vi "SubPanel_VIsList.vi"(8 "error in (no error)":errorcluster, 11 "SubPanelPath in":path) -> (0 "error out":errorcluster, 1 "SubP_VIsPathList":path[](array[path]), 2 "SubPanelsVis":string[](array[string]), 3 "SubPanelPath out":path)   [LabVIEW 2014, in "SubPanelModule.lvlib"]
uses:
  SubPanelModule.lvlib
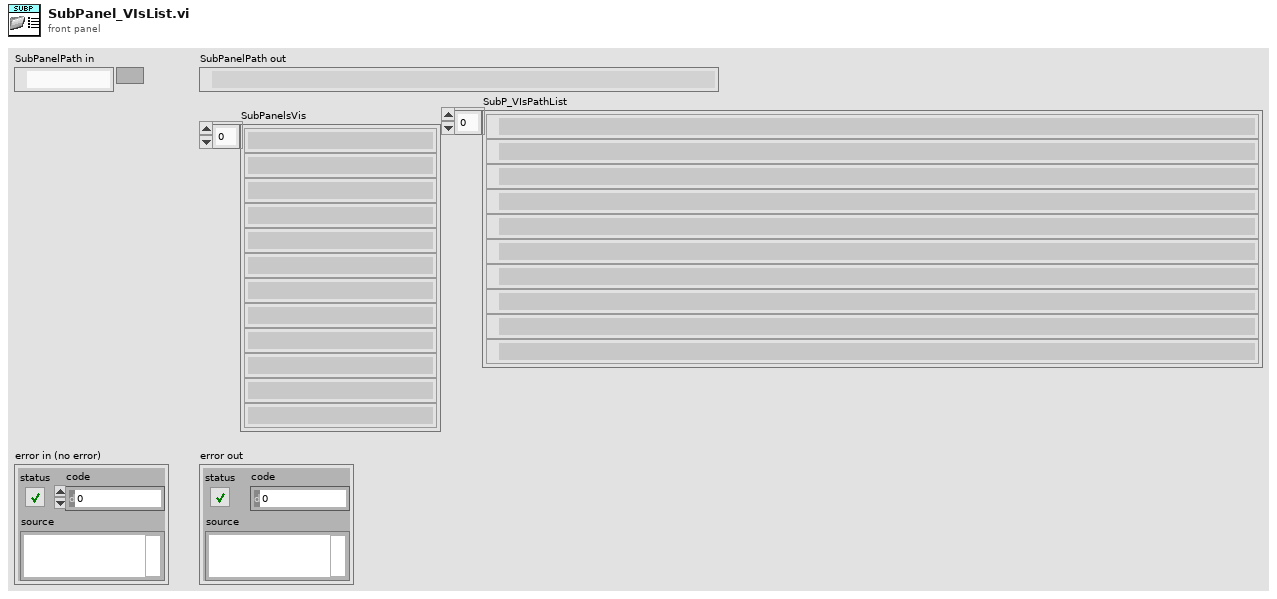
[diagram p1: front panel]
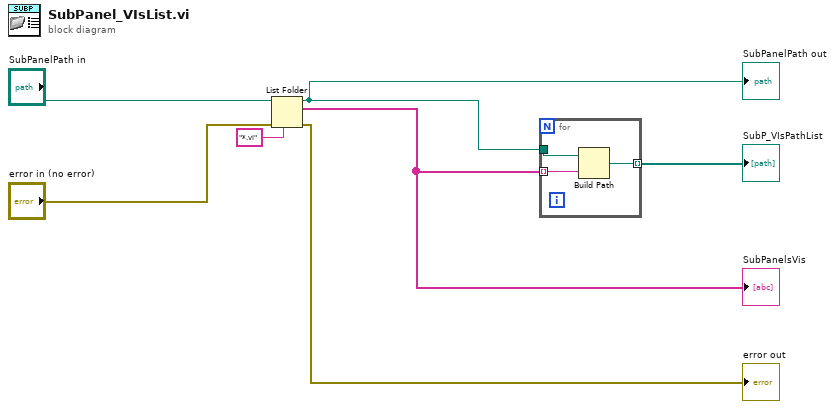
[diagram p0: block diagram]
diagram:
  n1 = List Folder(path="SubPanelPath in", pattern="*.vi", error in="error in (no error)") -> (path out=w3:path, filenames=w2:string[], error out=→"error out":errorcluster)  [unwired: 1 in, 1 out]
  "SubPanelsVis" <- w2
  "SubPanelPath out" <- w3
  n2 = for {
    tunnel: w3 -> [w10]
    tunnel: w2 -> [w9] mode=indexing
    tunnel: [w8] -> w1 mode=indexing
    n3 = Build Path(base path=w10, name or relative path=w9) -> (appended path=w8:path)
  }
  "SubP_VIsPathList" <- w1
